vi "Get Presets.vi"(1 "VISA Refnum in":refnum<visa-resource-name>, 6 "error in (no error)":errorcluster) -> (9 "read buffer":string, 13 "Wait":i32, 15 "Prescaler":i32, 17 "Trigger":i32, 19 "Threshold":i32, 21 "VISA Refnum out":refnum<visa-resource-name>, 26 "error out":errorcluster)   [LabVIEW 2012]
uses:
  <vilib>/Instr/_visa.llb/VISA Flush IO Buffer Mask.ctl
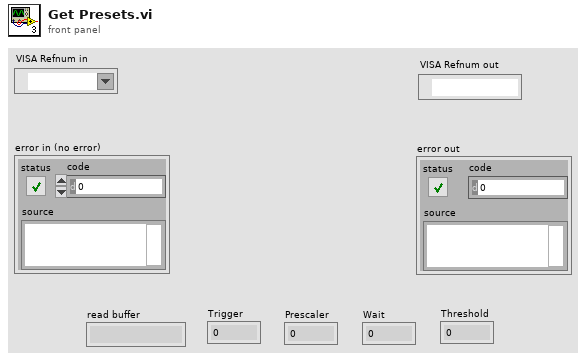
[diagram p1: front panel]
types:
  T1 = typedef "VISA Flush IO Buffer Mask.ctl" = u16
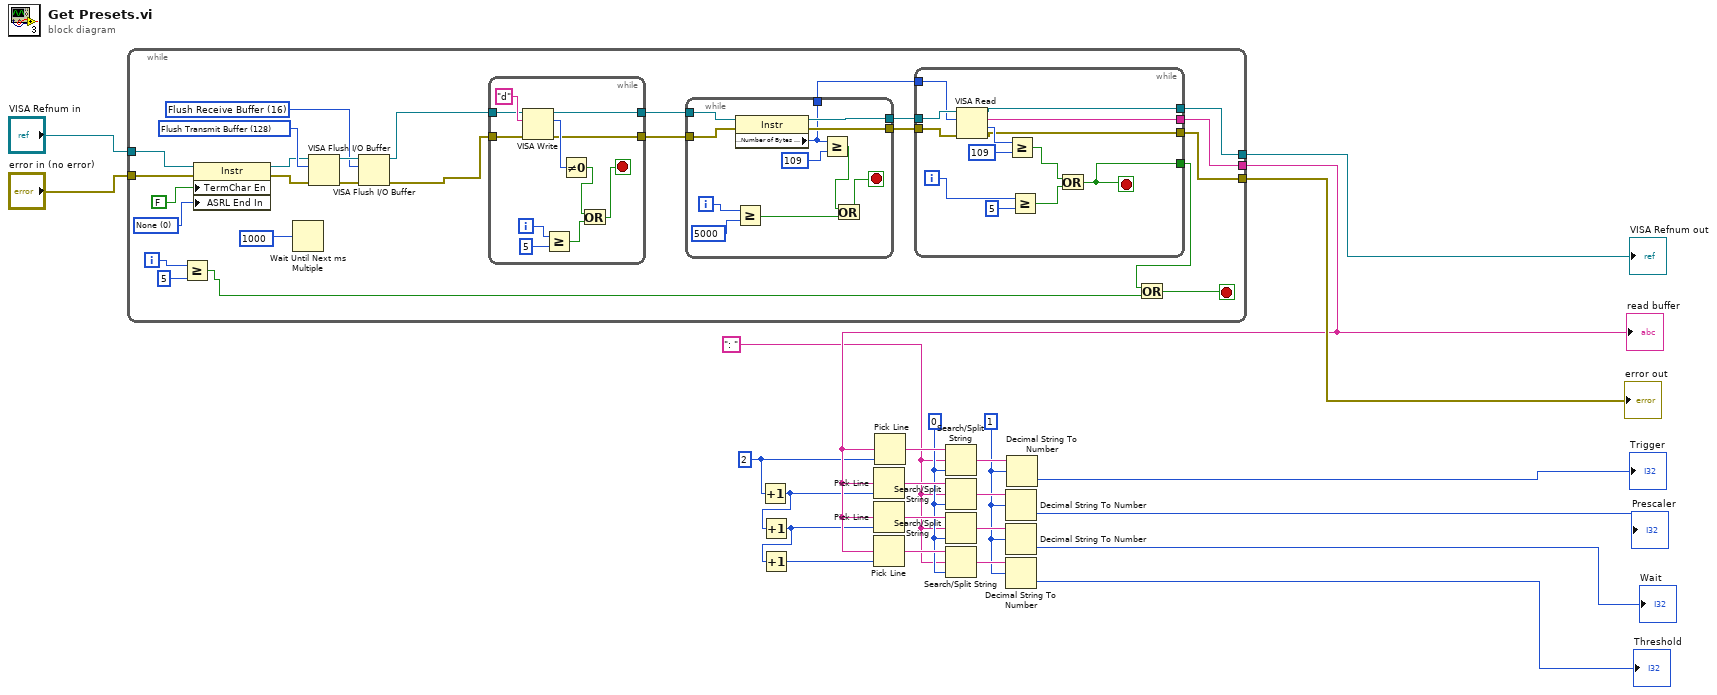
[diagram p0: block diagram]
diagram:
  w6 = 1 ("offset")
  w7 = 0 ("offset (0)")
  w5 = ": "
  w8 = 2 ("line index")
  n1 = while {
    tunnel: "VISA Refnum in" -> [w42]
    tunnel: "error in (no error)" -> [w43]
    tunnel: [w34] -> w22
    tunnel: [w33] -> w23
    tunnel: [w32] -> w24
    i -> [w31]
    stop <- w27 stop-if-true
    w44 = u16 0 items=["None", "Last Bit", "TermChar"] ("Serial Settings:End Mode for Reads")
    w47 = T1 16 items=["Flush Receive Buffer"=16, "Write Transmit Buffer to Device"=32, "Flush Receive Buffer (No I/O)"=64, "Flush Transmit Buffer"=128] ("Mask")
    w50 = T1 128 items=["Flush Receive Buffer"=16, "Write Transmit Buffer to Device"=32, "Flush Receive Buffer (No I/O)"=64, "Flush Transmit Buffer"=128] ("Mask")
    n2 = Greater Or Equal?(x=w31, y=5) -> (x >= y?=w28:bool)
    n3 = property class="Instr"(reference=w42, error in=w43, "TermChar En"=FALSE ("Message Based Settings:Termination Character Enable"), "ASRL End In"=w44) -> (reference out=w41:refnum<visa-resource-name>, error out=w40:errorcluster)
    n4 = Wait Until Next ms Multiple(millisecond multiple=u32 1000) -> ()  [unwired: 1 out]
    n5 = VISA Flush I/O Buffer(VISA resource name=w41, mask (16)=w50, error in (no error)=w40) -> (VISA resource name out=w49:refnum<visa-resource-name>, error out=w48:errorcluster)
    n6 = VISA Flush I/O Buffer(VISA resource name=w49, mask (16)=w47, error in (no error)=w48) -> (VISA resource name out=w26:refnum<visa-resource-name>, error out=w25:errorcluster)
    n7 = while {
      tunnel: w26 -> [w84]
      tunnel: w25 -> [w83]
      tunnel: [w81] -> w39
      tunnel: [w80] -> w38
      i -> [w78]
      stop <- w75 stop-if-true
      n8 = VISA Write(VISA resource name=w84, write buffer="d", error in (no error)=w83) -> (VISA resource name out=w81:refnum<visa-resource-name>, return count=w82:u32, error out=w80:errorcluster)
      n9 = Greater Or Equal?(x=w78, y=5) -> (x >= y?=w77:bool)
      n10 = Not Equal To 0?(x=w82) -> (x != 0?=w76:bool)
      n11 = Or(x=w76, y=w77) -> (x .or. y?=w75:bool)
    }
    n12 = while {
      tunnel: w39 -> [w73]
      tunnel: w38 -> [w72]
      tunnel: [w71] -> w37
      tunnel: [w70] -> w36
      tunnel: [w69] -> w35
      i -> [w68]
      stop <- w64 stop-if-true
      n13 = Greater Or Equal?(x=w68, y=5000) -> (x >= y?=w66:bool)
      n14 = property class="Instr"(reference=w73, error in=w72) -> (reference out=w71:refnum<visa-resource-name>, error out=w70:errorcluster, "Serial Settings:Number of Bytes at Serial Port"=w69:u32)
      n15 = Greater Or Equal?(x=w69, y=u32 109) -> (x >= y?=w65:bool)
      n16 = Or(x=w65, y=w66) -> (x .or. y?=w64:bool)
    }
    n17 = while {
      tunnel: w37 -> [w63]
      tunnel: w36 -> [w62]
      tunnel: w35 -> [w61]
      tunnel: [w58] -> w34
      tunnel: [w57] -> w33
      tunnel: [w56] -> w32
      tunnel: [w51] -> w29
      i -> [w55]
      stop <- w51 stop-if-true
      n18 = VISA Read(VISA resource name=w63, byte count=w61, error in (no error)=w62) -> (VISA resource name out=w57:refnum<visa-resource-name>, read buffer=w58:string, return count=w60:u32, error out=w56:errorcluster)
      n19 = Greater Or Equal?(x=w60, y=u32 109) -> (x >= y?=w53:bool)
      n20 = Greater Or Equal?(x=w55, y=5) -> (x >= y?=w52:bool)
      n21 = Or(x=w53, y=w52) -> (x .or. y?=w51:bool)
    }
    n22 = Or(x=w29, y=w28) -> (x .or. y?=w27:bool)
  }
  "error out" <- w24
  "VISA Refnum out" <- w23
  "read buffer" <- w22
  n23 = Increment(x=w8) -> (x+1=w11:i32)
  n24 = Increment(x=w11) -> (x+1=w10:i32)
  n25 = Increment(x=w10) -> (x+1=w9:i32)
  n26 = Pick Line(multi-line string=w22, line index=w11) -> (output string=w13:string)  [unwired: 1 in]
  n27 = Pick Line(multi-line string=w22, line index=w10) -> (output string=w14:string)  [unwired: 1 in]
  n28 = Pick Line(multi-line string=w22, line index=w9) -> (output string=w15:string)  [unwired: 1 in]
  n29 = Pick Line(multi-line string=w22, line index=w8) -> (output string=w12:string)  [unwired: 1 in]
  n30 = Search/Split String(string=w12, search string/char (-)=w5, offset (0)=w7) -> (match + rest of string=w16:string)  [unwired: 2 out]
  n31 = Search/Split String(string=w13, search string/char (-)=w5, offset (0)=w7) -> (match + rest of string=w17:string)  [unwired: 2 out]
  n32 = Search/Split String(string=w14, search string/char (-)=w5, offset (0)=w7) -> (match + rest of string=w18:string)  [unwired: 2 out]
  n33 = Search/Split String(string=w15, search string/char (-)=w5, offset (0)=w7) -> (match + rest of string=w19:string)  [unwired: 2 out]
  n34 = Decimal String To Number(string=w17, offset=w6) -> (number=→"Prescaler":i32)  [unwired: 1 in, 1 out]
  n35 = Decimal String To Number(string=w18, offset=w6) -> (number=→"Wait":i32)  [unwired: 1 in, 1 out]
  n36 = Decimal String To Number(string=w19, offset=w6) -> (number=→"Threshold":i32)  [unwired: 1 in, 1 out]
  n37 = Decimal String To Number(string=w16, offset=w6) -> (number=→"Trigger":i32)  [unwired: 1 in, 1 out]
